vi "Questionable Status Query.vi"(0 "VISA resource name":refnum<visa-resource-name>, 11 "error in (no error)":errorcluster) -> (4 "VISA resource name out":refnum<visa-resource-name>, 6 "Questionable Status":T1, 15 "error out":errorcluster)   [LabVIEW 2018, in "XP Power PLS600.lvlib"]
doc: "Returns the integer data explaining the questionable status monitored in the instrument.\n\nThe Questionable Status Register consists of the following 16 bits:\n\nBit 0: Over Voltage Error\nBit 1: Over Current Error\nBit 2: Reserved \nBit 3: Over Power Error\nBit 4: Temperature Error\nBit 5: Reserved \nBit 6: Reserved\nBit 7: Reserved\nBit 8: Not Calibrated\nBit 9: Hardware Error\nBit 10: Watchdog Error\nBit 11: Self-Test Error\nBit 12: Regulation Loss Error\nBit 13: Reserved\nBit 14: Reserved\nBit 15: Reserved"
uses:
  XP Power PLS600.lvlib
panel:
  # "Bit 0: Over Voltage Error\nBit 1: Over Current Error\nBit 2: Reserved\t\nBit 3: Over Power Error\nBit 4:\tTemperature Error\nBit 5: Reserved\t\nBit 6: Reserved\nBit 7: Reserved\nBit 8: Not Calibrated\nBit 9: Hardware Error\nBit 10: Watchdog Error\nBit 11: Self-Test Error\nBit 12: Regulation Loss Error\nBit 13: Reserved\nBit 14: Reserved\nBit 15: Reserved"
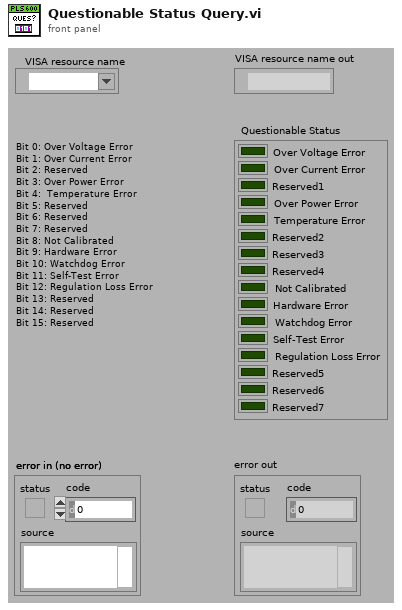
[diagram p1: front panel]
types:
  T1 = cluster{"Over Voltage Error":bool, "Over Current Error":bool, "Reserved1":bool, "Over Power Error":bool, "Temperature Error":bool, "Reserved2":bool, "Reserved3":bool, "Reserved4":bool, "Not Calibrated":bool, "Hardware Error":bool, "Watchdog Error":bool, "Self-Test Error":bool, "Regulation Loss Error":bool, "Reserved5":bool, "Reserved6":bool, "Reserved7":bool}
  T2 = cluster{"Operation Complete":bool, "Not Used":bool, "Query Error":bool, "Device Error":bool, "Message Available":bool, "Command Error":bool, "Not Used":bool, "Power On":bool, "Operation Complete 2":bool, "Not Used 2":bool, "Query Error 2":bool, "Device Error 2":bool, "Message Available 2":bool, "Command Error 2":bool, "Not Used 3":bool, "Not Used 4":bool}
  T3 = cluster{"Boolean array[0]":bool, "Boolean array[1]":bool, "Boolean array[2]":bool, "Boolean array[3]":bool, "Boolean array[4]":bool, "Boolean array[5]":bool, "Boolean array[6]":bool, "Boolean array[7]":bool, "Boolean array[8]":bool, "Boolean array[9]":bool, "Boolean array[10]":bool, "Boolean array[11]":bool, "Boolean array[12]":bool, "Boolean array[13]":bool, "Boolean array[14]":bool, "Boolean array[15]":bool}
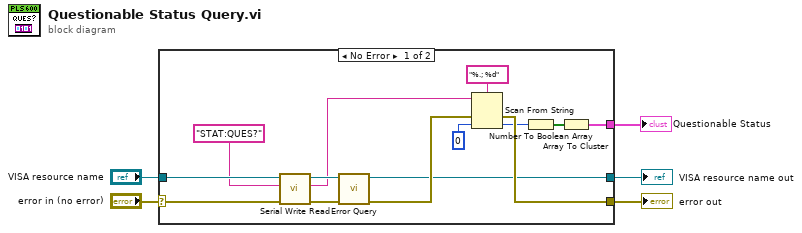
[diagram p0: block diagram]
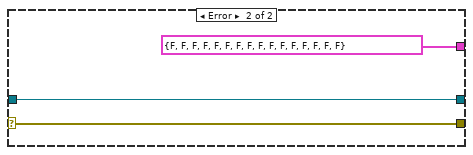
[diagram p2: hidden frame]
diagram:
  n1 = case shown="No Error" "error in (no error)" {
    selector: "error in (no error)" -> [w11 w22]
    tunnel: [w18 w22] -> w5
    tunnel: [w6 w21] -> w4
    tunnel: "VISA resource name" -> [w12 w21]
    tunnel: [w15 T2 {"Operation Complete"=FALSE, "Not Used"=FALSE, "Query Error"=FALSE, "Device Error"=FALSE, "Message Available"=FALSE, "Command Error"=FALSE, "Not Used"=FALSE, "Power On"=FALSE, "Operation Complete 2"=FALSE, "Not Used 2"=FALSE, "Query Error 2"=FALSE, "Device Error 2"=FALSE, "Message Available 2"=FALSE, "Command Error 2"=FALSE, "Not Used 3"=FALSE, "Not Used 4"=FALSE} ("Operation Status")] -> w1
    frame No Error {
      n2 = call "Serial Write Read.vi"("error in (no error)"=w11, "Write Buffer"="STAT:QUES?" ("Command to Send (empty)"), "VISA resource name"=w12) -> ("error out"=w9:errorcluster, "Read Buffer"=w8:string, "VISA resource name out"=w13:refnum<visa-resource-name>)  [unwired: 6 in]
      n3 = call "Error Query.vi"("error in (no error)"=w9, "VISA resource name"=w13) -> ("error out"=w7:errorcluster, "VISA resource name out"=w6:refnum<visa-resource-name>)  [unwired: 6 in, 2 out]
      n4 = Scan From String(format string="%.; %d" ("Format String"), input string=w8, error in=w7, default 1=u16 0 ("default value 1")) -> (error out=w18:errorcluster, output 1=w14:u16)  [unwired: 1 in, 2 out]
      n5 = Number To Boolean Array(number=w14) -> (Boolean array=w17:bool[])
      n6 = Array To Cluster(array=w17) -> (cluster=w15:T3)
    }
    frame Error {
    }
  }
  "error out" <- w5
  "VISA resource name out" <- w4
  "Questionable Status" <- w1
